vi "Time Stamp To FIle Name.vi"(7 "time format string (%c)":string="%Y%m%d%H%M%S", 10 "Time Stamp In":timestamp format="%<%.3X %x>T") -> (2 "File Name Out":string)   [LabVIEW 2024]
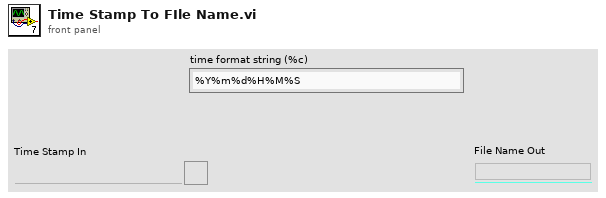
[diagram p1: front panel]
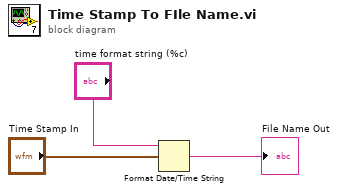
[diagram p0: block diagram]
diagram:
  n1 = Format Date/Time String(time format string (%c)="time format string (%c)", seconds (now)="Time Stamp In") -> (date/time string=→"File Name Out":string)  [unwired: 1 in]
